vi "To XML - Invalid character in Stack Trace - XML does not contain invalid character.vi"() -> ()   [LabVIEW 2013, in "JUnit XML Tests.lvlib" / "Test Case.lvlib"]
uses:
  Test Case.lvlib
  JUnit XML/Test Case/Test Case.lvclass
  <vilib>/xml/Close Reference(Node).vi
  <vilib>/addons/_JKI Toolkits/Caraya/classes/Assert/Assert Equal Value_Variant.vi
  <vilib>/addons/_JKI Toolkits/Caraya/classes/Test/Test.lvclass
  <vilib>/addons/_JKI Toolkits/Caraya/classes/Assert/Assert.lvclass
  <resource>/objmgr/DOMUserDefRef.rc
  <vilib>/xml/NI_XML.lvlib
panel:
  out "error out":errorcluster
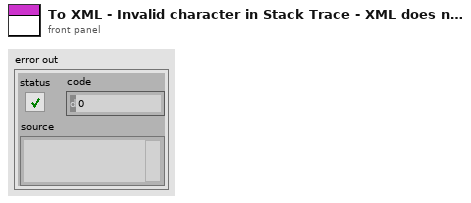
[diagram p1: front panel]
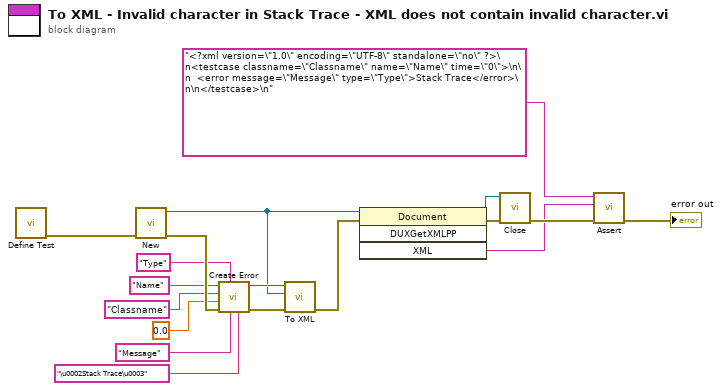
[diagram p0: block diagram]
diagram:
  n1 = call <vilib>:"Define Test.vi"() -> ("error out"=w18:errorcluster)  [unwired: 10 in, 1 out]
  n2 = call <vilib>:"New.vi"("error in (no error)"=w18) -> ("error out"=w15:errorcluster, "DOM document out"=w2:refnum<k20>)  [unwired: 7 in]
  n3 = call "Create Error.vi"("Stack Trace"="\u0002Stack Trace\u0003", "Message"="Message", "Type"="Type", "error in (no error)"=w15, "Time"=0.0, "Classname"="Classname", "Name"="Name") -> ("error out"=w16:errorcluster, "Test Case"=w17:refnum<class "Test Case.lvclass">)  [unwired: 3 in]
  n4 = call-dynamic "To XML.vi"("error in (no error)"=w16, "Parent"=w2, "Test Case in"=w17) -> ("error out"=w1:errorcluster)  [unwired: 8 in]
  n5 = invoke class="Document" method="DUXGetXMLPP"(reference=w2, error in=w1) -> (reference out=w13:refnum<k20>, error out=w14:errorcluster, "XML"=w11:string)  [unwired: 2 in, 1 out]
  n6 = call-poly <vilib>:"Close.vi"("error in (no error)"=w14, "node"=w13) -> ("error out"=w12:errorcluster)  [unwired: 7 in]
  n7 = call-poly <vilib>:"Assert.vi"("error in (no error)"=w12, "Actual"=w11, "Expected"="<?xml version=\"1.0\" encoding=\"UTF-8\" standalone=\"no\" ?>\n<testcase classname=\"Classname\" name=\"Name\" time=\"0\">\n\n  <error message=\"Message\" type=\"Type\">Stack Trace</error>\n\n</testcase>\n") -> ("error out"=→"error out":errorcluster)  [unwired: 7 in, 1 out]
